vi "CAN_LIN_Demo.vi"(11 "Sender":string="CAN_LIN_Demo0") -> ()   [LabVIEW 2014]
uses:
  <vilib>/Utility/miscctls.llb/LVPointTypeDef.ctl
  TSMaster_API/LIN_Function/Typedef/TSLIN_Transmit.ctl
  TSMaster_API/All_Control/Typedef/Hardware Type.ctl
  Utilities/Typedef/Hardware_Subtype.ctl
  TSMaster_API/CAN_CANFD_Function/Typedef/TSCAN_CAN_Configuration.ctl
  TSMaster_API/LIN_Function/Typedef/TSLIN_SetData.ctl
  TSMaster_API/LIN_Function/Typedef/TSLIN_LIN_Set.ctl
panel:
  out "error out":errorcluster
  in  "Config":bool
  in  "Connect":bool
  in  "Disconnect":bool
  out "Connect ?":bool
  in  "DLL_PATH":path=path "D:/Program Files (x86)/TOSUN/TSMaster/bin/TSMaster.dll"
  in  "选项卡控件":T1(tab)
  in  "CAN_Config_Array":T2[](array[typedef]) {"AAppChannel" items=["CHN1", "CHN2", "CHN3", "CHN4", "CHN5", "CHN6", "CHN7", "CHN8", "CHN9", "CHN10", "CHN11", "CHN12", "CHN13", "CHN14", "CHN15", "CHN16", "CHN17", "CHN18", "CHN19", "CHN20", "CHN21", "CHN22", "CHN23", "CHN24", "CHN25", "CHN26", "CHN27", "CHN28", "CHN29", "CHN30", "CHN31", "CHN32"]; "AHwChannel" items=["CHN1", "CHN2", "CHN3", "CHN4", "CHN5", "CHN6", "CHN7", "CHN8", "CHN9", "CHN10", "CHN11", "CHN12", "CHN13", "CHN14", "CHN15", "CHN16", "CHN17", "CHN18", "CHN19", "CHN20", "CHN21", "CHN22", "CHN23", "CHN24", "CHN25", "CHN26", "CHN27", "CHN28", "CHN29", "CHN30", "CHN31", "CHN32"]; "HardwareType" items=["BUS_UNKNOWN_TYPE", "TS_TCP_DEVICE", "XL_USB_DEVICE", "TS_USB_DEVICE", "PEAK_USB_DEVICE", "KVASER_USB_DEVICE", "ZLG_USB_DEVICE", "ICS_USB_DEVICE", "TS_TC1005_DEVICE", "CANABLE_USB_DEVICE", "TS_WIRELESS_OBD", "TS_USB_DEVICE_EX", "IXXAT_USB_DEVICE", "TS_ETH_IF_DEVICE", "TS_USB_IF_DEVICE", "BUS_DEV_TYPE_COUNT"]}
  in  "CAN_Channels used":u16(ring)=2 items=["1 Channel"=1, "2 Channels"=2, "3 Channels"=3, "4 Channels"=4, "5 Channels"=5, "6 Channels"=6, "7 Channels"=7, "8 Channels"=8, "9 Channels"=9, "10 Channels"=10, "11 Channels"=11, "12 Channels"=12, "13 Channels"=13, "14 Channels"=14, "15 Channels"=15, "16 Channels"=16]
  in  "LIN_Channels used":u16(ring)=1 items=["1 Channel"=1, "2 Channels"=2, "3 Channels"=3, "4 Channels"=4, "5 Channels"=5, "6 Channels"=6, "7 Channels"=7, "8 Channels"=8, "9 Channels"=9, "10 Channels"=10, "11 Channels"=11, "12 Channels"=12, "13 Channels"=13, "14 Channels"=14, "15 Channels"=15, "16 Channels"=16]
  in  "LIN_Data.LIN_Set_Array":T5[](array[typedef]) {"Set_node_funtiontype" items=["MasterNode", "SlaveNode", "MonitorNote"]; "Set"."Hardware Type" items=["BUS_UNKNOWN_TYPE", "TS_TCP_DEVICE", "XL_USB_DEVICE", "TS_USB_DEVICE", "PEAK_USB_DEVICE", "KVASER_USB_DEVICE", "ZLG_USB_DEVICE", "ICS_USB_DEVICE", "TS_TC1005_DEVICE", "CANABLE_USB_DEVICE", "TS_WIRELESS_OBD", "TS_USB_DEVICE_EX", "IXXAT_USB_DEVICE", "TS_ETH_IF_DEVICE", "TS_USB_IF_DEVICE", "BUS_DEV_TYPE_COUNT"]; "Set"."AHwChannel" items=["CHN1", "CHN2", "CHN3", "CHN4", "CHN5", "CHN6", "CHN7", "CHN8", "CHN9", "CHN10", "CHN11", "CHN12", "CHN13", "CHN14", "CHN15", "CHN16", "CHN17", "CHN18", "CHN19", "CHN20", "CHN21", "CHN22", "CHN23", "CHN24", "CHN25", "CHN26", "CHN27", "CHN28", "CHN29", "CHN30", "CHN31", "CHN32"]; "Set"."AAppChannel" items=["CHN1", "CHN2", "CHN3", "CHN4", "CHN5", "CHN6", "CHN7", "CHN8", "CHN9", "CHN10", "CHN11", "CHN12", "CHN13", "CHN14", "CHN15", "CHN16", "CHN17", "CHN18", "CHN19", "CHN20", "CHN21", "CHN22", "CHN23", "CHN24", "CHN25", "CHN26", "CHN27", "CHN28", "CHN29", "CHN30", "CHN31", "CHN32"]; "Set"."AProtocol" items=["Lin_Protocol_13", "Lin_Protocol_20", "Lin_Protocol_21", "Lin_Protocol_J2602"]}
  in  "LIN_Send":bool
  out "successful？":bool
  in  "loop send？":bool=TRUE
  out "Data":T7
  in  "Creat error":bool
  in  "log":i32(listbox)
  in  "Quit":bool
  # "CAN_LIN Demo"
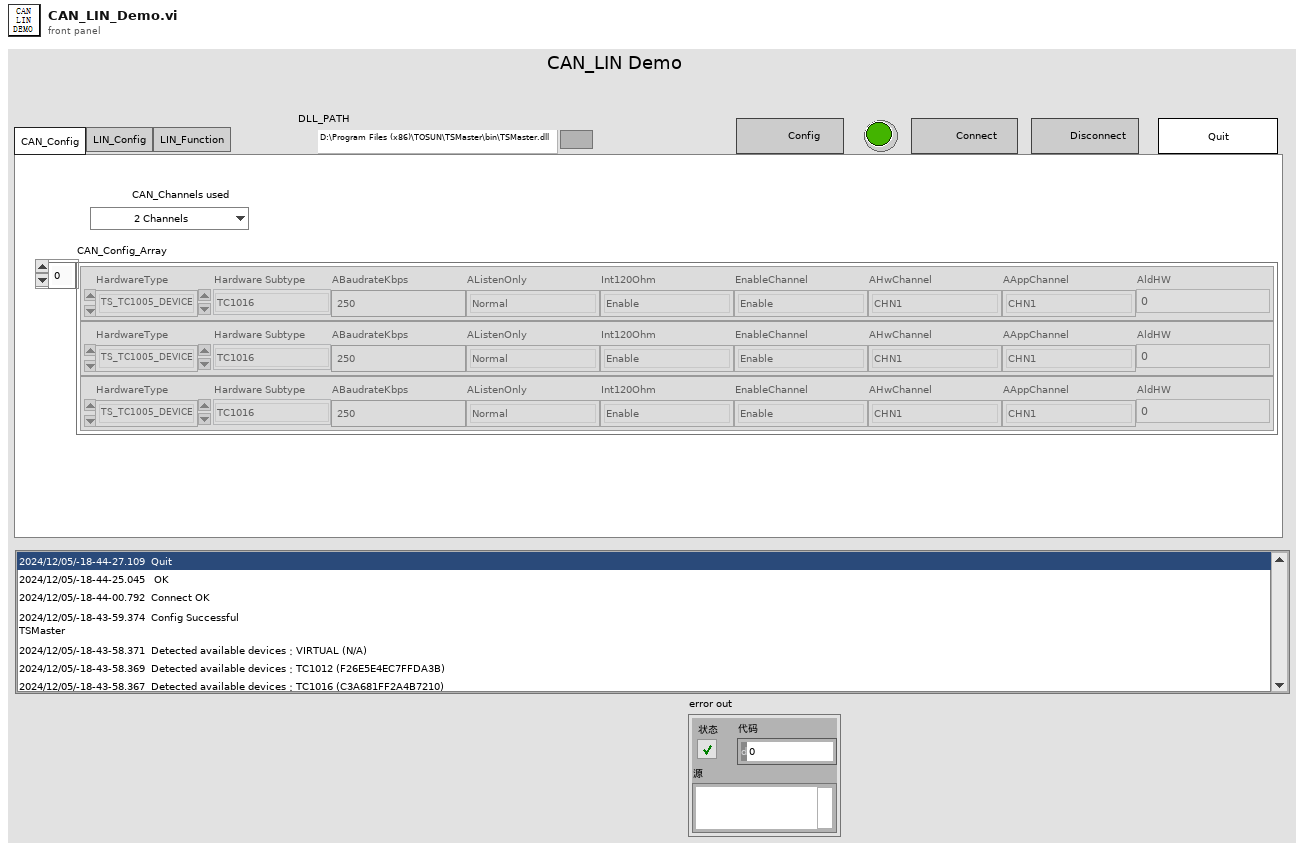
[diagram p1: front panel]
types:
  T1 = enum32{"CAN_Config", "LIN_Config", "LIN_Function"}
  T2 = typedef "TSCAN_CAN_Configuration.ctl" = cluster{"HardwareType":T3, "Hardware Subtype":T4, "ABaudrateKbps":sgl, "AListenOnly":enum16{"Normal", "ListenOnly"}, "Int120Ohm":enum16{"Disable", "Enable"}, "EnableChannel":enum16{"Disable", "Enable"}, "AHwChannel":i32, "AAppChannel":i32, "AldHW":i32}
  T3 = typedef "Hardware Type.ctl" = i32
  T4 = typedef "Hardware_Subtype.ctl" = enum16{"TS_UNKNOWN_DEVICE", "TSCAN_PRO", "TSCAN_Lite1", "TC1001", "TL1001", "TC1011", "TM5011", "TC1002", "TC1014", "TSCANFD2517", "TC1026", "TC1016", "TC1012", "TC1013", "TLog1002", "TC1034", "TC1018", "GW2116", "TC2115", "MP1013", "TC1113", "TC1114", "TP1013", "TC1017", "TP1018", "TF10XX", "TL1004_FD_4_LIN_2", "TE1051", "TP1051", "TP1034", "TTS9015", "TP1026", "TTS1026", "TTS1034", "TTS1018", "TL1011", "TTS1015_LiAuto", "TTS1013_LiAuto", "TTS1016Pro", "TC1054Pro", "TC1054", "TLog1038", "TO1013", "TC1034Pro", "TC1018Pro", "TC1038Pro", "TS_DEV_END"}
  T5 = typedef "TSLIN_LIN_Set.ctl" = cluster{"Set":T6, "Set_node_funtiontype":i32}
  T6 = typedef "TSLIN_SetData.ctl" = cluster{"Hardware Type":T3, "Hardware Subtype":T4, "AHwChannel":i32, "AAppChannel":i32, "ABaudrateKbps":sgl, "AProtocol":i32, "AldHW":i32}
  T7 = cluster{"Communication message":cluster{"Sender":string, "receiver":string, "message":string, "data":variant}, "Receive data":string, "error in":errorcluster}
  T8 = cluster{"Sender":string, "receiver":string, "message":string, "data":variant}
  T9 = enum8{"Enabled", "Disabled", "Disabled and Grayed Out"}
  T10 = typedef "LVPointTypeDef.ctl" = cluster{"Horizontal":i16, "Vertical":i16}
  T11 = cluster{"value0":u8, "value 1":u8, "value 2":u8, "value 3":u8, "value 4":u8, "value 5":u8, "value 6":u8, "value 7":u8}
  T12 = typedef "TSLIN_Transmit.ctl" = cluster{"Channel":i32, "Rx/TX":enum16{"Rx", "Tx"}, "Set_node_funtiontype":i32, "DLC":u32, "ID":u32, "FDatas":cluster{"value0":u8, "value 1":u8, "value 2":u8, "value 3":u8, "value 4":u8, "value 5":u8, "value 6":u8, "value 7":u8}}
  T13 = enum32{"invalid app kind", "Development System", "Run Time System", "Student Edition", "Embedded LabVIEW", "Evaluation", "Custom"}
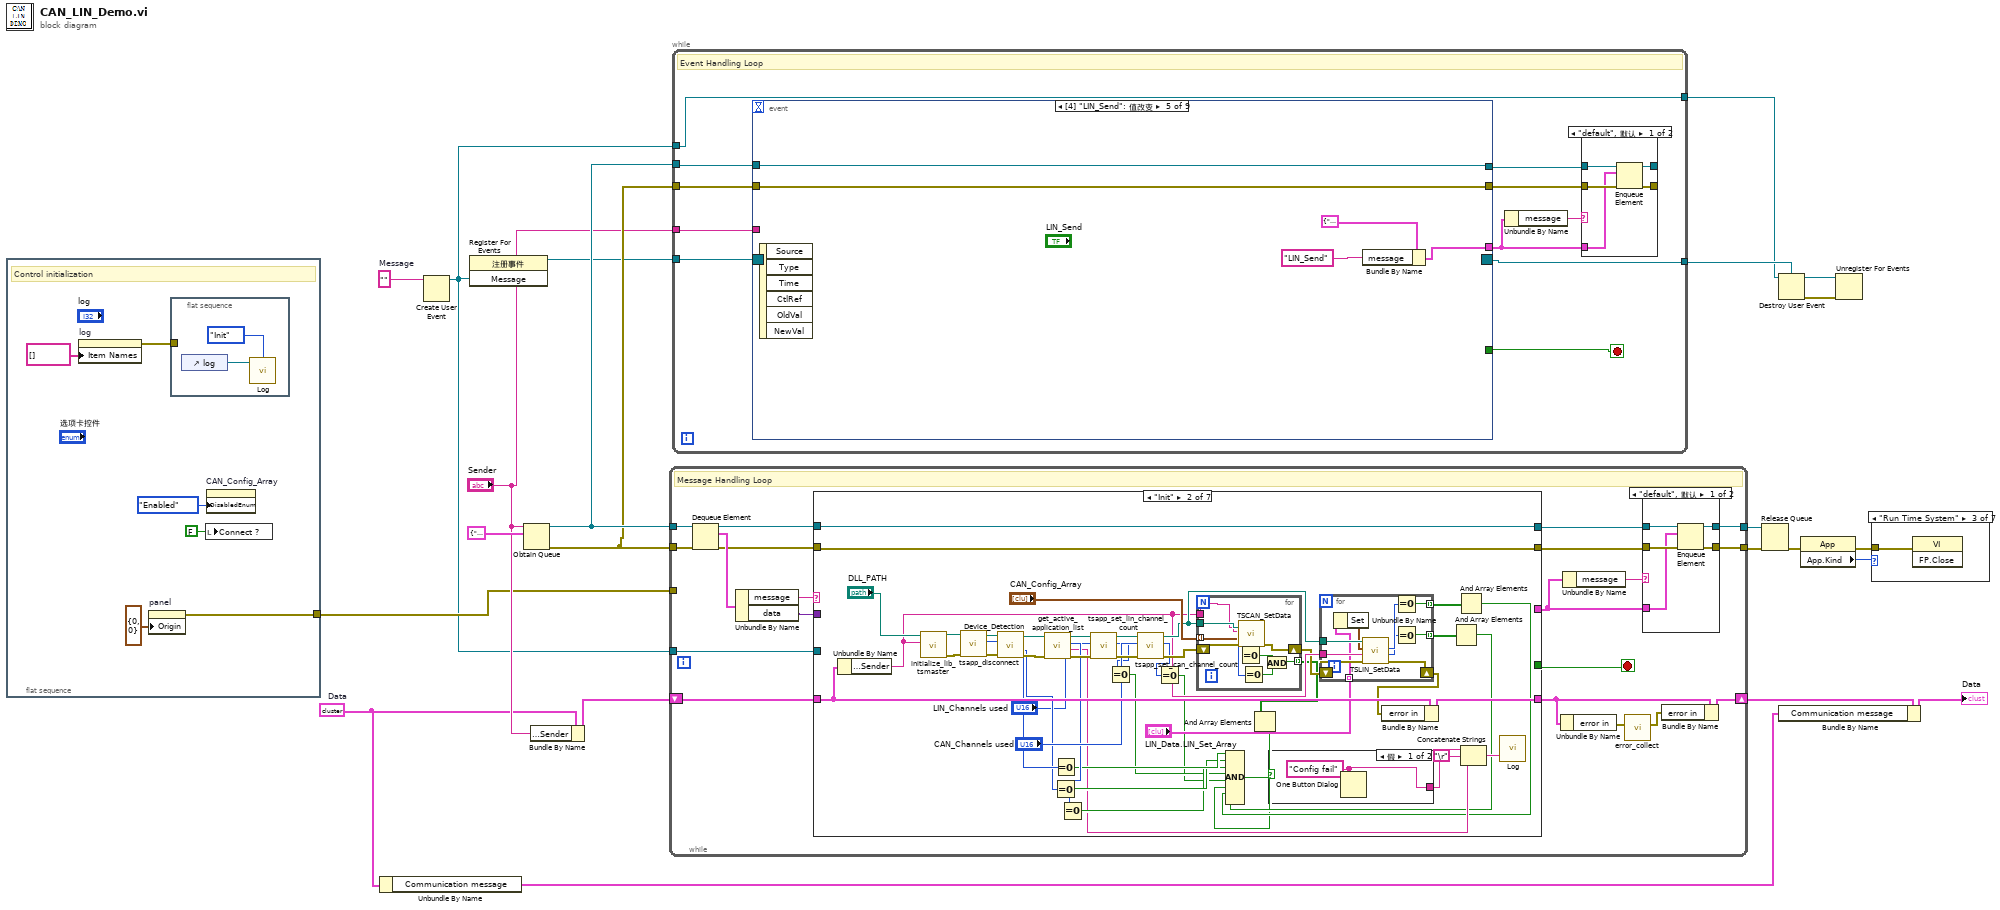
[diagram p0: block diagram]
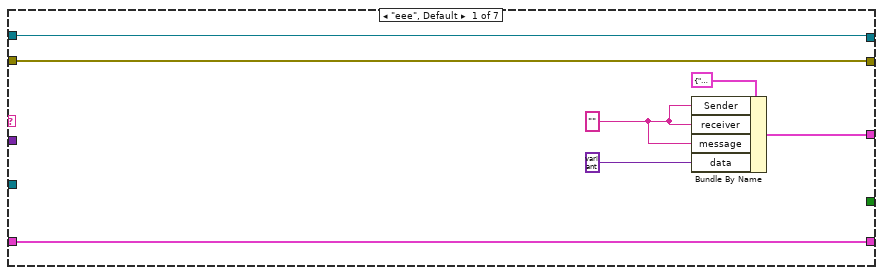
[diagram p9: hidden frame]
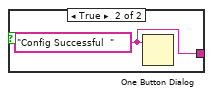
[diagram p10: hidden frame]
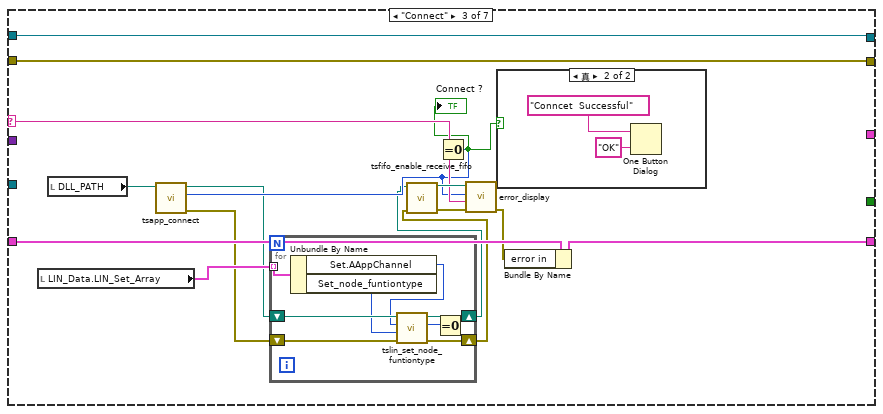
[diagram p11: hidden frame]
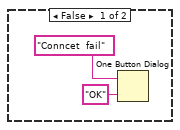
[diagram p12: hidden frame]
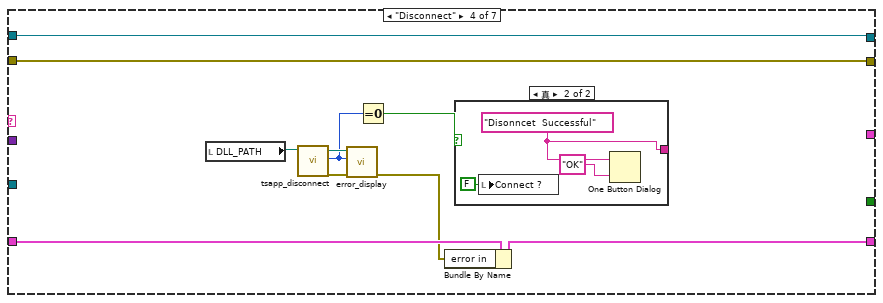
[diagram p13: hidden frame]
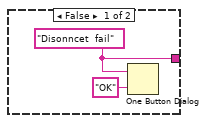
[diagram p14: hidden frame]
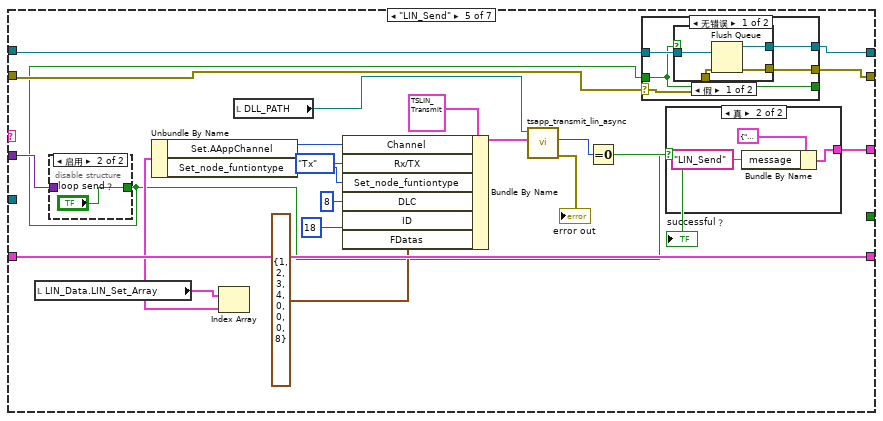
[diagram p15: hidden frame]
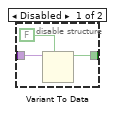
[diagram p16: hidden frame]
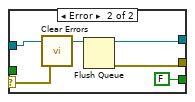
[diagram p19: hidden frame]
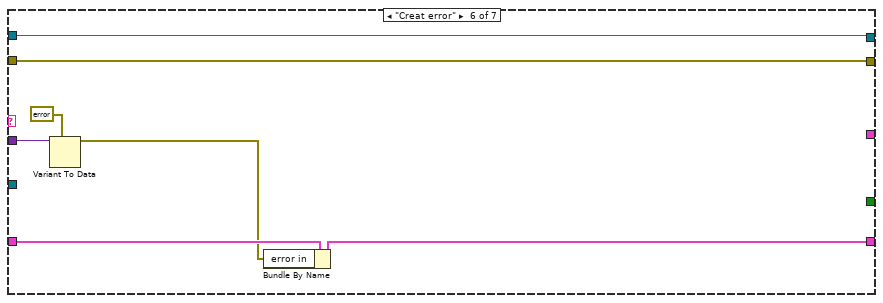
[diagram p20: hidden frame]
diagram:
  w11 = ""  # Message
  w3 = T7 {"Communication message"={"Sender"="", "receiver"="", "message"="", "data"=variant}, "Receive data"="", "error in"={"status"=FALSE, "code"=0, "source"=""}}  # Data
  n1 = flat-sequence {
    tunnel: [w26] -> w9
    frame #0 {
      # "Control initialization"
      n2 = property on="log" class="LstBox (严格)"("Item Names"=string[] [] ("项名")) -> (error out=w24:errorcluster)  [unwired: 2 in, 1 out]
      n3 = property on="panel" class="Pane"("Origin"=T10 {"Horizontal"=0, "Vertical"=0} ("原点")) -> (error out=w26:errorcluster)  [unwired: 2 in, 1 out]
      n4 = flat-sequence {
        tunnel: w24 -> [_]
        frame #0 {
          n5 = control-ref of="log"() -> (w28:refnum<vi>)
          n6 = call "Log.vi"("Method"=enum16{"Init", "Log"}."Init", "ListBox in"=w28) -> ()  [unwired: 2 in]
        }
      }
      n7 = local write "Connect ?"(FALSE ("Connect ?")) -> ()
      n8 = property on="CAN_Config_Array" class="Arr (严格)"("DisabledEnum"=T9."Enabled" ("禁用")) -> ()  [unwired: 2 in, 2 out]
    }
  }
  n9 = Unbundle By Name(w3) -> ("Communication message"=w1:T8)
  n10 = Create User Event(user event datatype=w11) -> (user event=w6:refnum<user-event>)  [unwired: 1 in, 1 out]
  n11 = register-events(w6) -> (reference out=w10:refnum<event-registration>)  [unwired: 2 in, 1 out]
  n12 = Obtain Queue(name (unnamed)="Sender", element data type=T8 {"Sender"="", "receiver"="", "message"="", "data"=variant} ("Communication message")) -> (queue out=w21:refnum<queue>, error out=w14:errorcluster)  [unwired: 3 in, 1 out]
  n13 = Bundle By Name(cluster=w3, "Communication message.Sender"="Sender") -> (w13:T7)
  n14 = while {
    tunnel: w21 -> [w49]
    tunnel: w14 -> [w48]
    tunnel: [w40] -> w20
    tunnel: [w39] -> w19
    shift-right: [w31] -> w4
    shift-left: w13 -> [w35]
    tunnel: w9 -> [_]
    tunnel: w6 -> [w34]
    stop <- w38 stop-if-true
    # "Message Handling Loop"
    n15 = Dequeue Element(queue=w49, error in (no error)=w48) -> (queue out=w45:refnum<queue>, element=w47:T8, error out=w44:errorcluster)  [unwired: 1 in, 1 out]
    n16 = Unbundle By Name(w47) -> ("message"=w46:string, "data"=w41:variant)
    n17 = case shown="\"Init\"" w46 {
      selector: w46 -> [_ _ w140 _ _ _ _]
      tunnel: [w63 w108 w146 w168 w189 w225 w232] -> w43
      tunnel: w45 -> [w63 w108 w146 w168 w190 w225 w231]
      tunnel: w44 -> [w62 w107 w145 w167 w187 w224 w229]
      tunnel: [w62 w107 w145 w167 w188 w224 w230] -> w42
      tunnel: w41 -> [_ _ _ _ w176 w222 _]
      tunnel: [_ _ _ _ _ _ TRUE] -> w38
      tunnel: [w60 _ _ _ w186 _ _] -> w37
      tunnel: [w57 w88 w139 w162 w195 w220 w228] -> w33
      tunnel: w35 -> [w57 w100 w144 w166 w195 w223 w228]
      tunnel: w34 -> [_ _ _ _ _ _ w227]
      frame "eee", Default {
        w58 = ""
        n18 = Bundle By Name(cluster=T8 {"Sender"="", "receiver"="", "message"="", "data"=variant} ("Communication message"), "Sender"=w58, "receiver"=w58, "message"=w58, "data"=variant) -> (w60:T8)
      }
      frame "Init" {
        n19 = Unbundle By Name(w100) -> ("Communication message.Sender"=w91:string)
        n20 = call "initialize_lib_tsmaster.vi"("AppName"=w91, "Path input"="DLL_PATH") -> ("error output"=w106:errorcluster, "Path output"=w101:path)  [unwired: 8 in]
        n21 = call "tsapp_disconnect.vi"("error in (no error)"=w106, "Path"=w101) -> ("error output"=w105:errorcluster, "retuen"=w82:i32, "Path output"=w102:path)  [unwired: 7 in]
        n22 = call "Device_Detection.vi"("error in (no error)"=w105, "Path"=w102) -> ("error out"=w104:errorcluster, "retuen"=w81:i32, "Path output"=w103:path)  [unwired: 7 in]
        n23 = call "get_active_application_list.vi"("error in"=w104, "path in"=w103) -> ("error out"=w96:errorcluster, "ATSMasterAppNames"=w70:string, "return"=w80:i32, "path out"=w97:path)  [unwired: 6 in]
        n24 = Equal To 0?(x=w81) -> (x = 0?=w76:bool)
        n25 = Equal To 0?(x=w82) -> (x = 0?=w77:bool)
        n26 = Equal To 0?(x=w80) -> (x = 0?=w75:bool)
        n27 = call "tsapp_set_lin_channel_count.vi"("error in (no error)"=w96, "Aount"="LIN_Channels used", "Path"=w97) -> ("error out"=w99:errorcluster, "return"=w79:i32, "Path output"=w98:path)  [unwired: 6 in]
        n28 = Equal To 0?(x=w79) -> (x = 0?=w74:bool)
        n29 = call "tsapp_set_can_channel_count.vi"("error in (no error)"=w99, "Aount"="CAN_Channels used", "Path"=w98) -> ("error out"=w93:errorcluster, "return"=w78:i32, "Path output"=w92:path)  [unwired: 6 in]
        n30 = Equal To 0?(x=w78) -> (x = 0?=w73:bool)
        n31 = for {
          tunnel: w92 -> [w130]
          tunnel: [w124] -> w72 mode=indexing
          tunnel: w91 -> [w123]
          tunnel: "CAN_Config_Array" -> [w122] mode=indexing
          shift-right: [w121] -> w89
          shift-left: w93 -> [w129]
          n32 = call "TSCAN_SetData.vi"("error in (no error)"=w129, "CAN configuration"=w122, "FAPppName"=w123, "Path"=w130) -> ("error out"=w121:errorcluster, "Config_retuen"=w127:i32, "maping_retuen"=w128:i32)  [unwired: 4 in, 1 out]
          n33 = Equal To 0?(x=w128) -> (x = 0?=w126:bool)
          n34 = Equal To 0?(x=w127) -> (x = 0?=w125:bool)
          n35 = And(x=w126, y=w125) -> (x .and. y?=w124:bool)
        }
        n36 = And Array Elements(Boolean array=w72) -> (logical AND=w66:bool)
        n37 = for {
          tunnel: w92 -> [w119]
          tunnel: [w115] -> w71 mode=indexing
          shift-right: [w118] -> w87
          shift-left: w89 -> [w120]
          tunnel: w91 -> [w114]
          tunnel: "LIN_Data.LIN_Set_Array" -> [w113] mode=indexing
          tunnel: [w111] -> w69 mode=indexing
          n38 = Unbundle By Name(w113) -> ("Set"=w112:T6)
          n39 = call "TSLIN_SetData.vi"("Error in"=w120, "AppName"=w114, "Set"=w112, "Path"=w119) -> ("Error out"=w118:errorcluster, "mapping_return"=w116:i32, "config_baud_return"=w117:i32)  [unwired: 4 in, 1 out]
          n40 = Equal To 0?(x=w117) -> (x = 0?=w115:bool)
          n41 = Equal To 0?(x=w116) -> (x = 0?=w111:bool)
        }
        n42 = Bundle By Name(cluster=w100, "error in"=w87) -> (w88:T7)
        n43 = And Array Elements(Boolean array=w69) -> (logical AND=w67:bool)
        n44 = And Array Elements(Boolean array=w71) -> (logical AND=w68:bool)
        n45 = Compound Arithmetic op=AND(w77, w76, w75, w74, w73, w66, w68, w67) -> (w65:bool)
        n46 = case shown="假" w65 {
          tunnel: [w109 w110] -> w86
          frame False {
            w109 = "Config fail" ("消息")
            n47 = One Button Dialog(message=w109) -> ()  [unwired: 1 in, 1 out]
          }
          frame True {
            w110 = "Config Successful  " ("消息")
            n48 = One Button Dialog(message=w110) -> ()  [unwired: 1 in, 1 out]
          }
        }
        n49 = Concatenate Strings(w86, "\r", w70) -> (w85:string)
        n50 = call "Log.vi"("Data"=w85) -> ()  [unwired: 3 in]
      }
      frame "Connect" {
        n51 = local read "LIN_Data.LIN_Set_Array"() -> (w135:T5[])
        n52 = local read "DLL_PATH"() -> (w143:path)
        n53 = call "tsapp_connect.vi"("Path"=w143) -> ("error out"=w132:errorcluster, "retuen"=w137:i32, "Path output"=w134:path)  [unwired: 8 in]
        n54 = for {
          shift-right: [w152] -> w133
          shift-left: w134 -> [w154]
          shift-right: [w151] -> w131
          shift-left: w132 -> [w153]
          tunnel: w135 -> [w150] mode=indexing
          n55 = Unbundle By Name(w150) -> ("Set.AAppChannel"=w149:i32, "Set_node_funtiontype"=w148:i32)
          n56 = call "tslin_set_node_funtiontype.vi"("错误输入（无错误）"=w153, "set_node_funtiontype"=w148, "AAppChannel"=w149, "path"=w154) -> ("错误输出"=w151:errorcluster, "return"=w147:i32, "path out"=w152:path)  [unwired: 5 in]
          n57 = Equal To 0?(x=w147) -> ()  [unwired: 1 out]
        }
        n58 = call "tsfifo_enable_receive_fifo.vi"("error in (no error)"=w131, "Path"=w133) -> ("error out"=w141:errorcluster, "Path output"=w142:path)  [unwired: 8 in]
        n59 = Equal To 0?(x=w137) -> (x = 0?=w136:bool)
        "Connect ?" <- w136
        n60 = call "error_display.vi"("error in"=w141, "Action name"=w140, "return"=w137, "DLL path"=w142) -> ("error out"=w138:errorcluster)  [unwired: 6 in, 1 out]
        n61 = case shown="真" w136 {
          frame False {
            n62 = One Button Dialog(message="Conncet  fail" ("消息"), button name ("OK")="OK" ("按钮名称（“确定”）")) -> ()  [unwired: 1 out]
          }
          frame True {
            n63 = One Button Dialog(message="Conncet  Successful" ("消息"), button name ("OK")="OK" ("按钮名称（“确定”）")) -> ()  [unwired: 1 out]
          }
        }
        n64 = Bundle By Name(cluster=w144, "error in"=w138) -> (w139:T7)
      }
      frame "Disconnect" {
        n65 = local read "DLL_PATH"() -> (w165:path)
        n66 = call "tsapp_disconnect.vi"("Path"=w165) -> ("error output"=w163:errorcluster, "retuen"=w160:i32, "Path output"=w164:path)  [unwired: 8 in]
        n67 = call "error_display.vi"("error in"=w163, "return"=w160, "DLL path"=w164) -> ("error out"=w161:errorcluster)  [unwired: 7 in, 1 out]
        n68 = Equal To 0?(x=w160) -> (x = 0?=w159:bool)
        n69 = Bundle By Name(cluster=w166, "error in"=w161) -> (w162:T7)
        n70 = case shown="真" w159 {
          tunnel: [w169 w172] -> _
          frame False {
            w169 = "Disonncet  fail" ("消息")
            n71 = One Button Dialog(message=w169, button name ("OK")="OK" ("按钮名称（“确定”）")) -> ()  [unwired: 1 out]
          }
          frame True {
            w172 = "Disonncet  Successful" ("消息")
            n72 = local write "Connect ?"(FALSE ("Connect ?")) -> ()
            n73 = One Button Dialog(message=w172, button name ("OK")="OK" ("按钮名称（“确定”）")) -> ()  [unwired: 1 out]
          }
        }
      }
      frame "LIN_Send" {
        n74 = local read "LIN_Data.LIN_Set_Array"() -> (w184:T5[])
        n75 = disable-structure shown="启用" {
          disable-tunnel: w176 -> [w197 _]
          disable-tunnel: [w196 "loop send？"] -> w175
          frame Disabled {
            n76 = Variant To Data(type=FALSE, Variant=w197) -> (data=w196:bool)  [unwired: 1 in, 1 out]
          }
          frame Enabled {
          }
        }
        n77 = Index Array(array=w184) -> (element=w183:T5)  [unwired: 1 in]
        n78 = Unbundle By Name(w183) -> ("Set.AAppChannel"=w182:i32, "Set_node_funtiontype"=w180:i32)
        n79 = local read "DLL_PATH"() -> (w191:path)
        n80 = Bundle By Name(cluster=T12 {"Channel"=0, "Rx/TX"=enum."Rx", "Set_node_funtiontype"=0, "DLC"=0, "ID"=0, "FDatas"={"value0"=0, "value 1"=0, "value 2"=0, "value 3"=0, "value 4"=0, "value 5"=0, "value 6"=0, "value 7"=0}} ("LIN_Transmit"), "Channel"=w182, "Rx/TX"=enum16{"Rx", "Tx"}."Tx", "Set_node_funtiontype"=w180, "DLC"=u32 8, "ID"=u32 18, "FDatas"=T11 {"value0"=1, "value 1"=2, "value 2"=3, "value 3"=4, "value 4"=0, "value 5"=0, "value 6"=0, "value 7"=8}) -> (w193:T12)
        n81 = call "tsapp_transmit_lin_async.vi"("LIN_Transmit"=w193, "Path"=w191) -> ("error out"=→"error out":errorcluster, "return"=w192:i32)  [unwired: 7 in, 1 out]
        n82 = Equal To 0?(x=w192) -> (x = 0?=→"successful？":bool)
        n83 = case shown="无错误" w187 {
          selector: w187 -> [w203 w217]
          tunnel: w175 -> [w204 _]
          tunnel: [w204 FALSE] -> _
          tunnel: w190 -> [w207 w216]
          tunnel: [w206 w215] -> w189
          tunnel: [w205 w214] -> w188
          frame No Error {
            n84 = case shown="假" w204 {
              tunnel: w207 -> [w211 w213]
              tunnel: [w210 w213] -> w206
              tunnel: [w209 w212] -> w205
              tunnel: w203 -> [w208 w212]
              frame False {
                n85 = Flush Queue(queue=w211, error in (no error)=w208) -> (queue out=w210:refnum<queue>, error out=w209:errorcluster)  [unwired: 1 out]
              }
              frame True {
              }
            }
          }
          frame Error {
            n86 = call <vilib>:"Clear Errors.vi"("error in (no error)"=w217) -> ()  [unwired: 5 in, 2 out]
            n87 = Flush Queue(queue=w216) -> (queue out=w215:refnum<queue>, error out=w214:errorcluster)  [unwired: 1 in, 1 out]
          }
        }
        n88 = case shown="真" w175 {
          tunnel: [_ w200] -> w186
          frame False {
          }
          frame True {
            n89 = Bundle By Name(cluster=T8 {"Sender"="", "receiver"="", "message"="", "data"=variant} ("Communication message"), "message"="LIN_Send") -> (w200:T8)
          }
        }
      }
      frame "Creat error" {
        n90 = Variant To Data(type=errorcluster {"status"=FALSE, "code"=0, "source"=""} ("error out"), Variant=w222) -> (data=w219:errorcluster)  [unwired: 1 in, 1 out]
        n91 = Bundle By Name(cluster=w223, "error in"=w219) -> (w220:T7)
      }
      frame "Quit" {
        w226 = "Quit" ("y")
        n92 = Generate User Event(user event=w227, event data cluster=w226) -> ()  [unwired: 2 in, 2 out]
        n93 = call "Log.vi"("Data"=w226) -> ()  [unwired: 3 in]
        n94 = Flush Queue(queue=w231, error in (no error)=w229) -> (queue out=w232:refnum<queue>, error out=w230:errorcluster)  [unwired: 1 out]
      }
    }
    n95 = Unbundle By Name(w33) -> ("error in"=w32:errorcluster)
    n96 = Unbundle By Name(w37) -> ("message"=w36:string)
    n97 = call "error_collect.vi"("error in (no error)"=w32) -> ("error IO"=w30:errorcluster)  [unwired: 10 in]
    n98 = case shown="\"default\", 默认" w36 {
      tunnel: w43 -> [w54 w56]
      tunnel: w42 -> [w53 w55]
      tunnel: w37 -> [w52 _]
      tunnel: [w51 w56] -> w40
      tunnel: [w50 w55] -> w39
      frame "default", Default {
        n99 = Enqueue Element(queue=w54, element=w52, error in (no error)=w53) -> (queue out=w51:refnum<queue>, error out=w50:errorcluster)  [unwired: 1 in, 1 out]
      }
      frame "" {
      }
    }
    n100 = Bundle By Name(cluster=w33, "error in"=w30) -> (w31:T7)
  }
  n101 = while {
    tunnel: w21 -> [w243]
    tunnel: w14 -> [w241]
    tunnel: "Sender" -> [w237]
    tunnel: w10 -> [w236]
    tunnel: [w235] -> w8
    tunnel: w6 -> [w234]
    tunnel: [w234] -> w5
    stop <- w244 stop-if-true
    # "Event Handling Loop"
    n102 = event shown="[4] \"LIN_Send\": 值改变" {
      selector: w236 -> [_ _ _ _ _ _ _ _ _]
      dyn-events: [_ _ _ _ _ _ _ _ _] -> w235
      timeout: _ -> [_ _ _ _ _ _ _ _ _]
      tunnel: [_ _ _ _ _ _ w281 w286 _] -> w244
      tunnel: w243 -> [w254 w259 w264 w269 w274 w279 w284 w289 w296]
      tunnel: [w254 w259 w264 w269 w274 w279 w284 w287 w296] -> w242
      tunnel: [T8 {"Sender"="", "receiver"="", "message"="", "data"=variant} ("Communication message") w255 w260 w265 w270 w277 _ _ w292] -> w239
      tunnel: [w253 w258 w263 w268 w273 w275 w280 w285 w295] -> w240
      tunnel: w241 -> [w253 w258 w263 w268 w273 w275 w280 w285 w295]
      tunnel: w237 -> [_ _ _ _ _ _ _ _ _]
      event Timeout {
        n103 = event-data() -> ()  [unwired: 1 in, 3 out]
      }
      event "Config": Value Change {
        n104 = event-data() -> ()  [unwired: 1 in, 6 out]
        n105 = Bundle By Name(cluster=T8 {"Sender"="", "receiver"="", "message"="", "data"=variant} ("Communication message"), "message"="Init") -> (w255:T8)
      }
      event "Connect": Value Change {
        n106 = event-data() -> ()  [unwired: 1 in, 6 out]
        n107 = Bundle By Name(cluster=T8 {"Sender"="", "receiver"="", "message"="", "data"=variant} ("Communication message"), "message"="Connect") -> (w260:T8)
      }
      event "Disconnect": Value Change {
        n108 = event-data() -> ()  [unwired: 1 in, 6 out]
        n109 = Bundle By Name(cluster=T8 {"Sender"="", "receiver"="", "message"="", "data"=variant} ("Communication message"), "message"="Disconnect") -> (w265:T8)
      }
      event "LIN_Send": Value Change {
        n110 = event-data() -> ()  [unwired: 1 in, 6 out]
        n111 = Bundle By Name(cluster=T8 {"Sender"="", "receiver"="", "message"="", "data"=variant} ("Communication message"), "message"="LIN_Send") -> (w270:T8)
      }
      event "Quit": Value Change {
        n112 = event-data() -> ()  [unwired: 1 in, 6 out]
        n113 = Bundle By Name(cluster=T8 {"Sender"="", "receiver"="", "message"="", "data"=variant} ("Communication message"), "message"="Quit" ("Sender")) -> (w277:T8)
      }
      event User Event {
        n114 = event-data() -> ("Message"=w283:string)  [unwired: 1 in]
        n115 = Equal?(x=w283, y="Quit") -> (x = y?=w281:bool)
      }
      event Panel Close? {
        w286 = TRUE ("放弃？")
        n116 = event-data() -> ()  [unwired: 1 in, 4 out]
        n117 = Enqueue Element(queue=w289, element=T8 {"Sender"="", "receiver"="", "message"="Quit", "data"=variant} ("Communication message")) -> (queue out=w287:refnum<queue>)  [unwired: 2 in, 2 out]
        n118 = event-data("Discard?"=w286) -> ()  [unwired: 1 in, 1 out]
      }
      event "Creat error": Value Change {
        n119 = event-data() -> ()  [unwired: 1 in, 6 out]
        n120 = To Variant(anything=errorcluster {"status"=TRUE, "code"=709394, "source"="This is a error demo"}) -> (Variant=w290:variant)
        n121 = Bundle By Name(cluster=T8 {"Sender"="", "receiver"="", "message"="", "data"=variant} ("Communication message"), "message"="Creat error" ("Sender"), "data"=w290) -> (w292:T8)
      }
    }
    n122 = Unbundle By Name(w239) -> ("message"=w238:string)
    n123 = case shown="\"default\", 默认" w238 {
      tunnel: w242 -> [w249 w251]
      tunnel: w240 -> [w248 w250]
      tunnel: w239 -> [w247 _]
      tunnel: [w246 w251] -> _
      tunnel: [w245 w250] -> _
      frame "default", Default {
        n124 = Enqueue Element(queue=w249, element=w247, error in (no error)=w248) -> (queue out=w246:refnum<queue>, error out=w245:errorcluster)  [unwired: 1 in, 1 out]
      }
      frame "" {
      }
    }
  }
  n125 = Release Queue(queue=w20, error in (no error)=w19) -> (error out=w18:errorcluster)  [unwired: 1 in, 2 out]
  n126 = Destroy User Event(user event=w5) -> (error out=w7:errorcluster)  [unwired: 1 in]
  n127 = Bundle By Name(cluster=w4, "Communication message"=w1) -> (→"Data":T7)
  n128 = property class="App"(error in=w18) -> (error out=w17:errorcluster, "App.Kind"=w16:T13)  [unwired: 1 in, 1 out]
  n129 = Unregister For Events(event registration refnum=w8, error in=w7) -> ()  [unwired: 1 out]
  n130 = case shown="\"Run Time System\"" w16 {
    tunnel: w17 -> [_ _ w297 _ _ _ _]
    frame "invalid app kind", Default {
    }
    frame "Development System" {
    }
    frame "Run Time System" {
      n131 = invoke class="VI" method="FP.Close"(error in=w297) -> ()  [unwired: 2 in, 3 out]
    }
    frame "Student Edition" {
    }
    frame "Embedded LabVIEW" {
    }
    frame "Evaluation" {
    }
    frame "Custom" {
    }
  }
